vi "sub_tcp_data_send.vi"(11 "packet data":string) -> (3 "read packet":string)   [LabVIEW 2019]
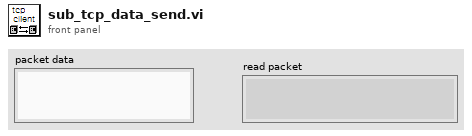
[diagram p1: front panel]
types:
  T1 = enum16{"Standard", "Buffered", "CRLF", "Immediate"}
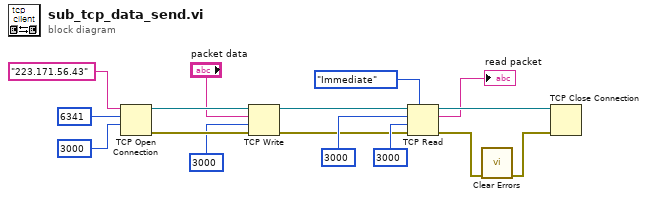
[diagram p0: block diagram]
diagram:
  n1 = TCP Open Connection(address="223.171.56.43" ("Machine"), remote port or service name=u16 6341 ("Port"), timeout ms (60000)=3000 ("타임아웃 ms (60000)")) -> (connection ID=w9:refnum<k5>, error out=w4:errorcluster)  [unwired: 1 in, 1 out]
  n2 = TCP Write(connection ID=w9, data in="packet data", error in (no error)=w4, 9:3000 ("타임아웃 ms (25000)")) -> (connection ID out=w6:refnum<k5>, error out=w5:errorcluster)  [unwired: 1 out]
  n3 = TCP Read(connection ID=w6, bytes to read=3000, error in (no error)=w5, 7:T1."Immediate" ("mode (standard)"), 9:3000 ("timeout ms (25000)")) -> (connection ID out=w10:refnum<k5>, data out=→"read packet":string, error out=w11:errorcluster)
  n4 = call <vilib>:"Clear Errors.vi"("error in (no error)"=w11) -> ("error out"=w7:errorcluster)  [unwired: 5 in, 1 out]
  n5 = TCP Close Connection(connection ID=w10, error in (no error)=w7) -> ()  [unwired: 1 in, 2 out]
